vi "Store-Recall Instrument State.vi"(7 "State Identification ( )":path, 8 "error in (no error)":errorcluster, 9 "Operation (0: Save State)":T1(ring), 11 "VISA resource name":refnum<visa-resource-name>) -> (0 "error out":errorcluster, 3 "VISA resource name out":refnum<visa-resource-name>)   [LabVIEW 2011, in "Agilent E5052X.lvlib"]
doc: "Stores, recalls or deletes a selected instrument state."
uses:
  Agilent E5052X.lvlib
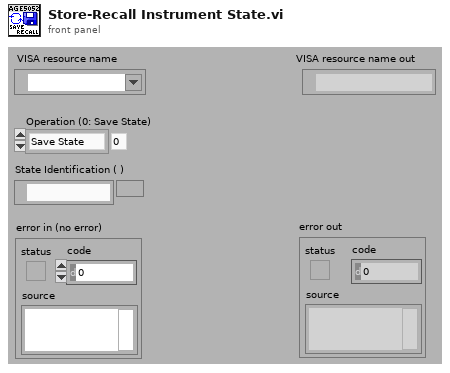
[diagram p1: front panel]
types:
  T1 = enum16{"Save State", "Recall State", "Delete State"}
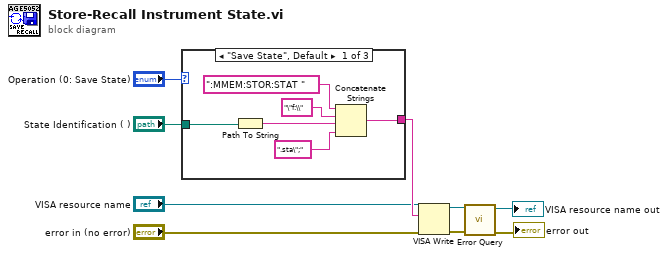
[diagram p0: block diagram]
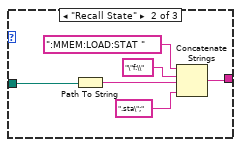
[diagram p2: hidden frame]
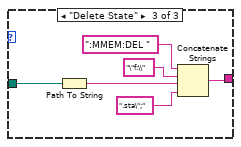
[diagram p3: hidden frame]
diagram:
  n1 = case shown="\"Save State\", Default" "Operation (0: Save State)" {
    tunnel: "State Identification ( )" -> [w11 w17 w23]
    tunnel: [w14 w18 w24] -> w7
    frame "Save State", Default {
      n2 = Path To String(path=w11) -> (string=w10:string)
      n3 = Concatenate Strings(":MMEM:STOR:STAT ", "\"f:\\", w10, ".sta\";") -> (w14:string)
    }
    frame "Recall State" {
      n4 = Path To String(path=w17) -> (string=w16:string)
      n5 = Concatenate Strings(":MMEM:LOAD:STAT ", "\"f:\\", w16, ".sta\";") -> (w18:string)
    }
    frame "Delete State" {
      n6 = Path To String(path=w23) -> (string=w22:string)
      n7 = Concatenate Strings(":MMEM:DEL ", "\"f:\\", w22, ".sta\";") -> (w24:string)
    }
  }
  n8 = VISA Write(VISA resource name="VISA resource name", write buffer=w7, error in (no error)="error in (no error)") -> (VISA resource name out=w6:refnum<visa-resource-name>, error out=w5:errorcluster)  [unwired: 1 out]
  n9 = call "Error Query.vi"("error in (no error)"=w5, "VISA resource name"=w6) -> ("error out"=→"error out":errorcluster, "VISA resource name out"=→"VISA resource name out":refnum<visa-resource-name>)  [unwired: 6 in, 2 out]
